vi "Last Ack.vi"(7 "Sender":refnum<class "Sender.lvclass">, 10 "Actor":refnum<class "Actor.lvclass">, 11 "TEMPLATE Actor in":refnum<class "TEMPLATE Actor.lvclass">) -> (3 "TEMPLATE Actor out":refnum<class "TEMPLATE Actor.lvclass">)   [LabVIEW 2020, in "_Template.lvlib" / "Templates.lvlib" / "TEMPLATE Actor.lvlib" / "TEMPLATE Actor.lvclass"]
uses:
  TEMPLATE Actor.lvclass
  jettl/jettl/Actor/Actor/Actor.lvclass
  jettl/jettl/Sender/Sender/Sender.lvclass
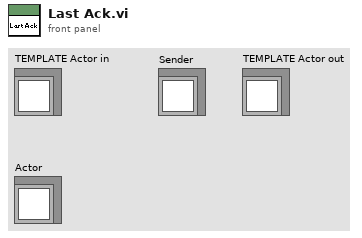
[diagram p1: front panel]
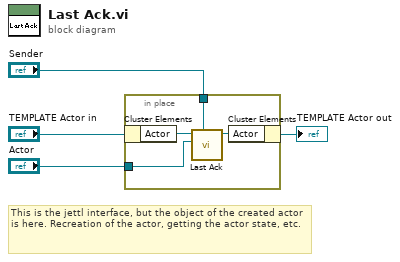
[diagram p0: block diagram]
diagram:
  # "This is the jettl interface, but the object of the created actor is here. Recreation of the actor, getting the actor state, etc."
  n1 = in-place {
    in-place-border: "Sender" -> [w6]
    in-place-border: "Actor" -> [w5]
    n2 = in-place-cluster #1("TEMPLATE Actor in") -> ("Actor"=w8:refnum<class "Actor.lvclass">)
    n3 = call-dynamic "Last Ack.vi"("Sender"=w6, "Actor"=w5, "Last Ack in"=w8) -> ("Last Ack out"=w7:refnum<class "Actor.lvclass">)  [unwired: 8 in]
    n4 = in-place-cluster #1("Actor"=w7) -> (→"TEMPLATE Actor out":refnum<class "TEMPLATE Actor.lvclass">)
  }
